vi "Flatten Names (Device).vi"(0 "names in":refnum<k21>[](array[refnum]), 11 "error in (no error)":errorcluster) -> (4 "names out":refnum<k21>, 15 "error out":errorcluster)   [LabVIEW 2020, in "SLSC.lvlib"]
doc: "Converts an array of device names into a comma-delimited list of device names. Example: [\"Mod1\",\"Mod2\",\"Mod3\"] -> \"Mod1,Mod2,Mod3\"."
uses:
  <vilib>/SLSC/SLSC.lvlib
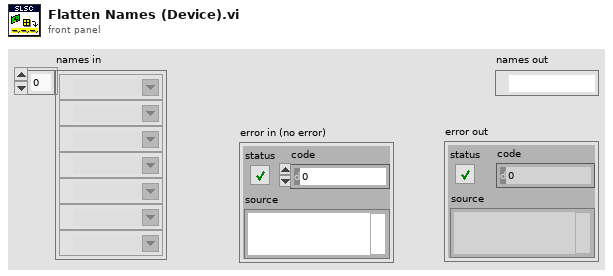
[diagram p1: front panel]
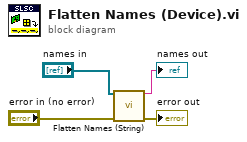
[diagram p0: block diagram]
diagram:
  n1 = call <vilib>:"Flatten Names (String).vi"("names in"="names in", "error in (no error)"="error in (no error)") -> ("names out"=→"names out":string, "error out"=→"error out":errorcluster)  [unwired: 12 in]
